vi "Error Converter (ErrCode or Status).vi"(8 "error in (no error)":errorcluster, 11 "error code":i32) -> (0 "error out":errorcluster)   [LabVIEW 2021, in "Olasdwf.lvlib"]
uses:
  Olasdwf.lvlib
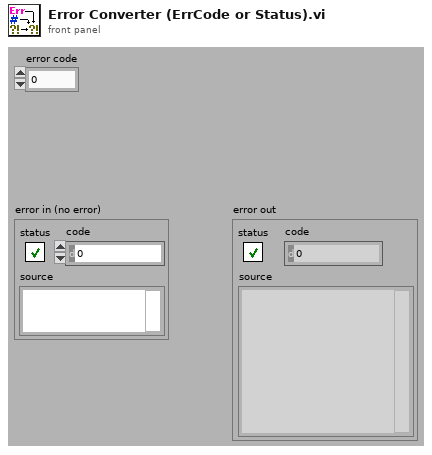
[diagram p1: front panel]
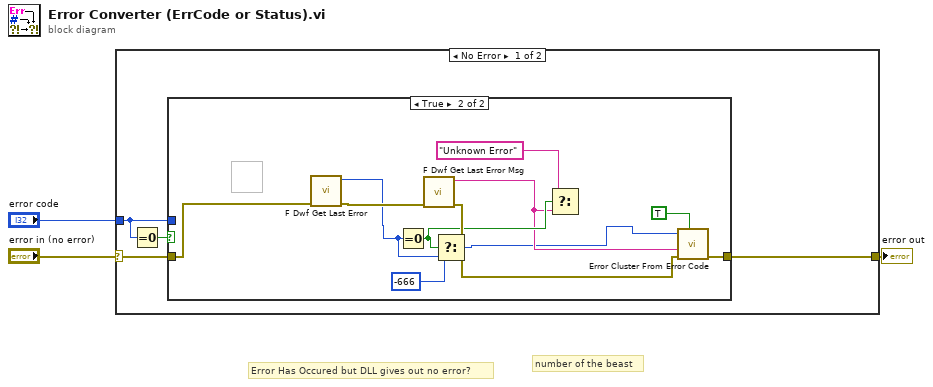
[diagram p0: block diagram]
diagram:
  # "number of the beast"
  # "Error Has Occured but DLL gives out no error?"
  n1 = case shown="No Error" "error in (no error)" {
    selector: "error in (no error)" -> [w6 w20]
    tunnel: [w4 w20] -> w2
    tunnel: "error code" -> [w5 _]
    frame No Error {
      n2 = Equal To 0?(x=w5) -> (x = 0?=w7:bool)
      n3 = case shown="True" w7 {
        tunnel: w6 -> [w8 w15]
        tunnel: w5 -> [_ _]
        tunnel: [w8 w19] -> w4
        frame False {
        }
        frame True {
          n4 = call "F Dwf Get Last Error.vi"("error in (no error)"=w15) -> ("error out"=w16:errorcluster, "pdwferc out"=w10:i32)  [unwired: 8 in, 1 out]
          n5 = Equal To 0?(x=w10) -> (x = 0?=w13:bool)
          n6 = call "F Dwf Get Last Error Msg.vi"("error in (no error)"=w16) -> ("error out"=w17:errorcluster, "szError out"=w12:string)  [unwired: 8 in, 1 out]
          n7 = Select(t=-666, s=w13, f=w10) -> (s? t:f=w9:i32)
          n8 = Select(t="Unknown Error", s=w13, f=w12) -> ()  [unwired: 1 out]
          n9 = call <vilib>:"Error Cluster From Error Code.vi"("show call chain? (False)"=TRUE, "error in (no error)"=w17, "error message (\"\")"=w12, "error code (0)"=w9) -> ("error out"=w19:errorcluster)  [unwired: 5 in]
        }
      }
    }
    frame Error {
    }
  }
  "error out" <- w2
